vi "DIOSerialTxLoop.vi"(11 "DIOSerialPortSettings":T1={"TxPort"="ModbusPort1Tx", "TxDataFIFO"="ModbusPort1TxFIFO", "TxHealthAndStatusFIFO"="ModbusPort1TxHealthAndStatusFIFO", "RxPort"="ModbusPort1Rx", "RxDataFIFO"="ModbusPort1RxFIFO", "RxHealthAndStatusFIFO"="ModbusPort1RxHealthAndStatusFIFO", "BaseHealthAndStatusAddress"=0, "TimestampRegister"="TimestampRegister", "TxTimestampFIFO"="ModbusPort1TimestampFIFO"}) -> ()   [LabVIEW 2016, in "FPGADIOSerialASCII.lvlib"]
uses:
  FPGADIOSerialASCII.lvlib
  DataTypes/DIOSerialPortSettings.ctl
  DataTypes/DIOSerialTxLoopData.ctl
  DataTypes/DIOSerialTxStates.ctl
  <vilib>/Platform/TimedLoop/XDataNode/timing_clust.ctl
  <vilib>/Platform/TimedLoop/XDataNode/nitl_modes.ctl
  <vilib>/Platform/TimedLoop/XDataNode/wakeup.ctl
  ts_M1M3Support/FPGA/Common_FPGA_HealthAndStatus/DataTypes/HealthAndStatusUpdateMode.ctl
  <vilib>/rvi/Emulation/niFpgaSctlEmulationGetInTimedLoop.vi
  <vilib>/rvi/Emulation/niFpgaEmulationReportErrorSimple.vi
  <vilib>/rvi/Emulation/niFpgaGetClockAttributes.vi
  <vilib>/rvi/Emulation/niFpgaCriticalErrorInLSC.vi
  <vilib>/rvi/DataTransferAndStorage/Container/Common/niFpgaContainerExecOnDevCompGetState.vi
  <vilib>/rvi/Emulation/niFpgaEmulationIsFPGAContextNoSignature.vi
  <vilib>/rvi/errors/niFpgaSetErrorForExecOnDevCompSimple.vi
  <vilib>/rvi/eio/common/nirviEmuReportErrorAndStop.vi
  <vilib>/rvi/DataTransferAndStorage/Container/Common/niFpgaContainerGetUniqueNameForEmu.vi
  <vilib>/rvi/FIFO/Fifo_Resource/nirvififoEmulationSetSize.vi
  <vilib>/rvi/FIFO/Fifo_Resource/nirviFifoEmulationQueueMgr.vi
  <instcachedir>/0/nirviFifoEmulationQueueMgr_E5CAEC123FF24DC58D834DCA3CDAA9B5.lvgen/nirviFifoEmulationQueueMgr_E5CAEC123FF24DC58D834DCA3CDAA9B5_002.vi
  <vilib>/rvi/FIFO/Fifo_Resource/nirvififoEmulationDetermineInputValidOut.vi
  <vilib>/rvi/FIFO/Fifo_Resource/nirvififoEmulationCreateLock.vi
  <vilib>/rvi/Emulation/niFpgaProcessEmulError.vi
  <vilib>/rvi/FIFO/Fifo_Resource/nirvififoEmulationObtainLock.vi
  <vilib>/rvi/FIFO/Fifo_Resource/nirvififoEmulationReleaseLock.vi
  <vilib>/rvi/occurrence/nirviWaitOnOccurrenceBase.vi
  <vilib>/rvi/errors/nirviReportUnexpectedCaseInternalError.vi
  <vilib>/rvi/errors/nirviReportUnexpectedCaseInternalError (U32).vi
  <vilib>/Utility/error.llb/Clear Errors.vi
  <vilib>/rvi/interface/RandomDataEmulation/niFpgaRandomDataHandleErrors.vi
  <vilib>/rvi/eio/common/nirviEmuTemplateMethod_errors.vi
  <vilib>/Platform/TimedLoop/XDataNode/XDataNode.xnode
  <vilib>/rvi/DataTransferAndStorage/Container/XNode/niFpgaContainer.xnode
  <vilib>/rvi/FIFO/Fifo_Resource/niFpgaFifoEmulationRefIn.vi
  <vilib>/eio/EIONode/EIONode.xnode
  ts_M1M3Support/FPGA/Common_FPGA_HealthAndStatus/FPGAHealthAndStatus.lvlib
  <vilib>/Platform/TimedLoop/XDataNode/XDNodeRunTimeDep.lvlib
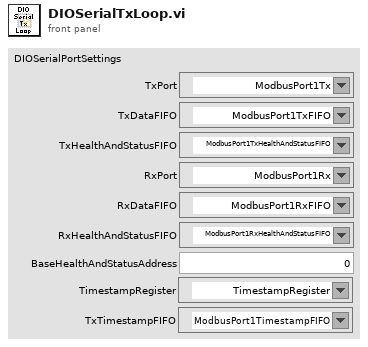
[diagram p1: front panel]
types:
  T1 = typedef "FPGADIOSerialASCII.lvlib/DIOSerialPortSettings.ctl" = cluster{"TxPort":refnum<k21>, "TxDataFIFO":refnum<k21>, "TxHealthAndStatusFIFO":refnum<k21>, "RxPort":refnum<k21>, "RxDataFIFO":refnum<k21>, "RxHealthAndStatusFIFO":refnum<k21>, "BaseHealthAndStatusAddress":u32, "TimestampRegister":refnum<k21>, "TxTimestampFIFO":refnum<k21>}
  T2 = typedef "FPGADIOSerialASCII.lvlib/DIOSerialTxLoopData.ctl" = cluster{"State":T3, "WriteData":u16, "DelayTicks":u32, "StateAfterDelay":T3, "Bit":u16, "BytesSent":u16}
  T3 = typedef "FPGADIOSerialASCII.lvlib/DIOSerialTxStates.ctl" = enum16{"GetByte", "Delay", "WriteBits"}
  T4 = typedef "XDNodeRunTimeDep.lvlib/timing_clust.ctl" = cluster{"Expected End [f-1]":u64, "Actual End [f-1]":u64, "Finished Late? [f-1]":bool, "Expected End [i-1]":u64, "Actual End [i-1]":u64, "Finished Late? [i-1]":bool, "Expected Start [i]":u64, "Actual Start [i]":u64, "Expected Start [f]":u64, "Actual Start [f]":u64, "Source Name":string, "Structure Name":string, "Period":i64, "Deadline":i64, "Offset":i64, "Start":i64, "Priority":i32, "Timeout":i32, "Mode":T5, "Wakeup Reason":T6, "Error":errorcluster, "Source Type":string, "Secondary Source Type":string, "Global End Time":u64, "Global Start Time":u64, "Frame Duration":u64, "Iteration Duration":u64, "Assigned CPU":i32, "I/O Scan Engine Mode":u32}
  T5 = typedef "XDNodeRunTimeDep.lvlib/nitl_modes.ctl" = enum32{"No Change", "Process missed periods, maintain original phase", "Discard missed periods, maintain original phase", "Process missed periods, ignore original phase", "Discard missed periods, ignore original phase"}
  T6 = typedef "XDNodeRunTimeDep.lvlib/wakeup.ctl" = enum32{"Normal", "Aborted", "Asynchronous wakeup", "Timing source error", "Timed loop error", "Timeout"}
  T7 = typedef "FPGAHealthAndStatus.lvlib/HealthAndStatusUpdateMode.ctl" = enum8{"NOP", "Set", "Add", "Subtract", "Or"}
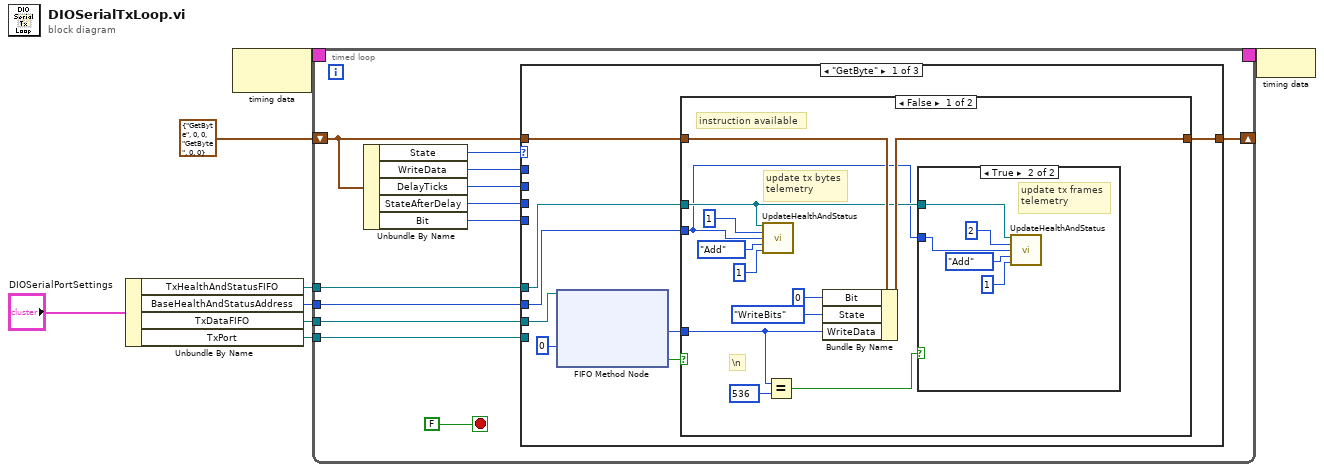
[diagram p0: block diagram]
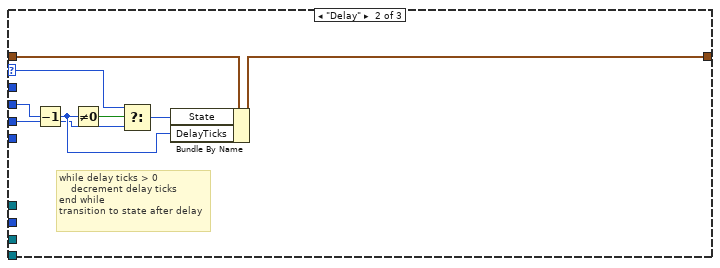
[diagram p4: hidden frame]
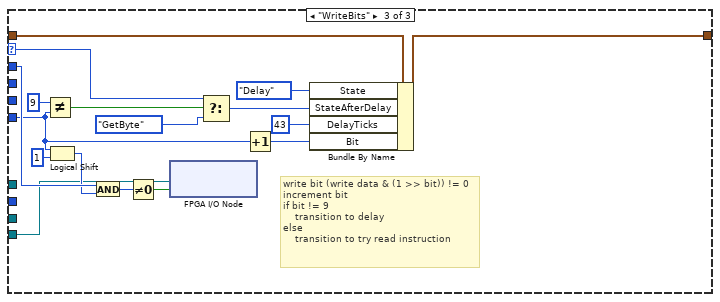
[diagram p5: hidden frame]
diagram:
  n1 = Unbundle By Name("DIOSerialPortSettings") -> ("TxHealthAndStatusFIFO"=w3:refnum<k21>, "BaseHealthAndStatusAddress"=w4:u32, "TxDataFIFO"=w5:refnum<k21>, "TxPort"=w6:refnum<k21>)
  n2 = node-c288() -> (w8:T4)  [unwired: 1 in]
  n3 = timed-loop {
    shift-right: [w20] -> _
    shift-left: T2 {"State"=enum."GetByte", "WriteData"=0, "DelayTicks"=0, "StateAfterDelay"=enum."GetByte", "Bit"=0, "BytesSent"=0} ("ModbusTxLoop") -> [w19]
    tunnel: w4 -> [w14]
    tunnel: w3 -> [w12]
    timing: w8 -> [_]
    timing-out: [_] -> w7
    tunnel: w5 -> [w11]
    tunnel: w6 -> [w10]
    stop <- FALSE stop-if-true
    n4 = Unbundle By Name(w19) -> ("State"=w18:T3, "WriteData"=w17:u16, "DelayTicks"=w16:u32, "StateAfterDelay"=w15:T3, "Bit"=w13:u16)
    n5 = case shown="\"GetByte\"" w18 {
      selector: w18 -> [_ w50 w65]
      tunnel: w19 -> [w28 w54 w68]
      tunnel: [w27 w53 w63] -> w20
      tunnel: w17 -> [_ _ w70]
      tunnel: w16 -> [_ w52 _]
      tunnel: w15 -> [_ w47 _]
      tunnel: w14 -> [w26 _ _]
      tunnel: w13 -> [_ _ w58]
      tunnel: w12 -> [w25 _ _]
      tunnel: w11 -> [w24 _ _]
      tunnel: w10 -> [_ _ w55]
      frame "GetByte" {
        n6 = xnode ("FIFO Method Node")("Timeout"=0, "FIFO In"=w24) -> ("Element"=w21:u16, "Timed Out?"=w22:bool)  [unwired: 1 out]
        n7 = case shown="False" w22 {
          tunnel: w21 -> [w33 _]
          tunnel: w28 -> [w40 w46]
          tunnel: [w39 w46] -> w27
          tunnel: w26 -> [w30 _]
          tunnel: w25 -> [w31 _]
          frame False {
            # "\\n"
            # "update tx bytes\ntelemetry"
            # "instruction available"
            # "instruction available"
            n8 = call "UpdateHealthAndStatus.vi"("InternalHealthAndStatusFIFO"=w31, "AddressOffset"=u32 1 ("x"), "BaseAddress"=w30, "HealthAndStatusUpdateMode"=HealthAndStatusUpdateMode."Add" ("Telemetry Update Mode"), "Data"=u64 1) -> ()  [unwired: 11 in]
            n9 = Equal?(x=w33, y=u16 536 ("Data")) -> (x = y?=w29:bool)
            n10 = Bundle By Name(cluster=w40, "Bit"=u16 0, "State"=DIOSerialTxStates."WriteBits", "WriteData"=w33) -> (w39:T2)
            n11 = case shown="True" w29 {
              tunnel: w31 -> [_ w42]
              tunnel: w30 -> [_ w43]
              frame False {
              }
              frame True {
                # "update tx frames\ntelemetry"
                n12 = call "UpdateHealthAndStatus.vi"("InternalHealthAndStatusFIFO"=w42, "AddressOffset"=u32 2 ("x"), "BaseAddress"=w43, "HealthAndStatusUpdateMode"=HealthAndStatusUpdateMode."Add" ("Telemetry Update Mode"), "Data"=u64 1) -> ()  [unwired: 11 in]
              }
            }
          }
          frame True {
            # "no instruction available"
            # "no instruction available"
          }
        }
      }
      frame "Delay" {
        # "while delay ticks > 0\n    decrement delay ticks\nend while\ntransition to state after delay"
        n13 = Decrement(x=w52) -> (x-1=w48:u32)
        n14 = Not Equal To 0?(x=w48) -> (x != 0?=w51:bool)
        n15 = Select(t=w50, s=w51, f=w47) -> (s? t:f=w49:T3)
        n16 = Bundle By Name(cluster=w54, "State"=w49, "DelayTicks"=w48) -> (w53:T2)
      }
      frame "WriteBits" {
        # "write bit (write data & (1 >> bit)) != 0\nincrement bit\nif bit != 9\n    transition to delay\nelse\n    transition to try read instruction"
        n17 = Not Equal?(x=u16 9, y=w58) -> (x != y?=w57:bool)
        n18 = Logical Shift(y=w58, x=u16 1) -> (x << y=w60:u16)
        n19 = And(x=w70, y=w60) -> (x .and. y?=w71:u16)
        n20 = Not Equal To 0?(x=w71) -> (x != 0?=w69:bool)
        n21 = xnode "FPGA I/O Node"("I/O Item"=w69, "FPGA I/O In"=w55) -> ()  [unwired: 1 out]
        n22 = Select(t=w65, s=w57, f=DIOSerialTxStates."GetByte" ("TransmitStates")) -> (s? t:f=w67:T3)
        n23 = Increment(x=w58) -> (x+1=w62:u16)
        n24 = Bundle By Name(cluster=w68, "State"=DIOSerialTxStates."Delay" ("TransmitStates"), "StateAfterDelay"=w67, "DelayTicks"=u16 43 ("Delay Ticks"), "Bit"=w62) -> (w63:T2)
      }
    }
  }
  n25 = node-c288(w7) -> ()
